vi "Prepare image to send.vi"(8 "error in (no error)":errorcluster, 10 "Image in":u16[][](array[numeric]), 11 "DAQOrcaFlash in":refnum<class "DAQOrcaFlash.lvclass">) -> (0 "error out":errorcluster, 2 "Data out":variant[](array[variant]), 3 "DAQOrcaFlash out":refnum<class "DAQOrcaFlash.lvclass">)   [LabVIEW 2012, in "DAQOrcaFlash.lvclass"]
uses:
  DAQOrcaFlash.lvclass
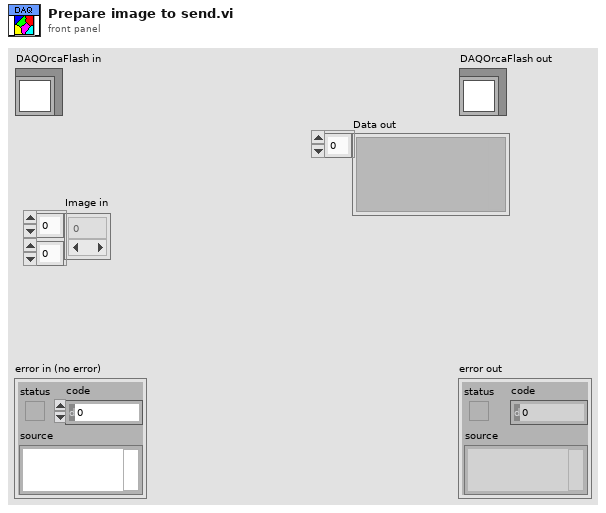
[diagram p1: front panel]
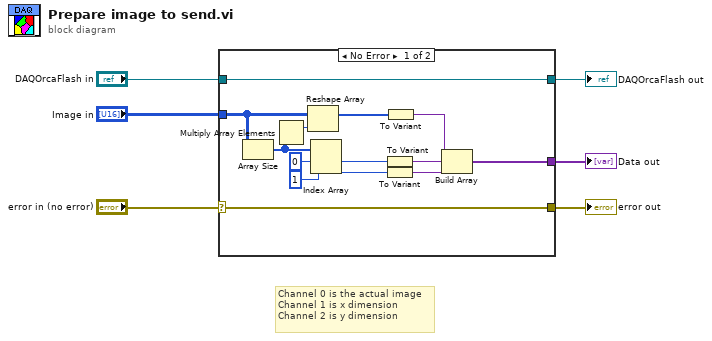
[diagram p0: block diagram]
diagram:
  # "Channel 0 is the actual image\nChannel 1 is x dimension\nChannel 2 is y dimension"
  n1 = case shown="No Error" "error in (no error)" {
    selector: "error in (no error)" -> [w19 w22]
    tunnel: [w19 w22] -> w5
    tunnel: [w20 w21] -> w3
    tunnel: "DAQOrcaFlash in" -> [w20 w21]
    tunnel: "Image in" -> [w16 _]
    tunnel: [w10 _] -> w1
    frame No Error {
      n2 = Array Size(array=w16) -> (size(s)=w8:i32[])
      n3 = Multiply Array Elements(1:w8) -> (0:w7:i32)
      n4 = Reshape Array(w16, w7) -> (w9:u16[])
      n5 = Index Array(array=w8, index #1=0 ("index"), index #2=1 ("index")) -> (element #1=w15:i32, element #2=w14:i32)
      n6 = To Variant(anything=w15) -> (Variant=w12:variant)
      n7 = To Variant(anything=w14) -> (Variant=w13:variant)
      n8 = To Variant(anything=w9) -> (Variant=w11:variant)
      n9 = Build Array(w11, w12, w13) -> (w10:variant[])
    }
    frame Error {
    }
  }
  "error out" <- w5
  "DAQOrcaFlash out" <- w3
  "Data out" <- w1
